vi "SUB_WriteFileAppendText_AnyFolder.vi"(2 "Input Text":string, 3 "Filename":string, 4 "base path":path) -> ()   [LabVIEW 2011]
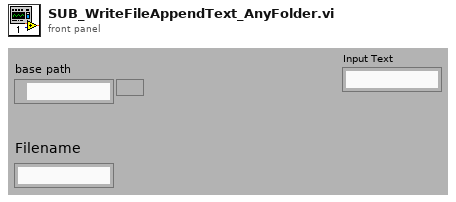
[diagram p1: front panel]
types:
  T1 = enum16{"open", "open or create", "create or replace", "create", "open (read only)"}
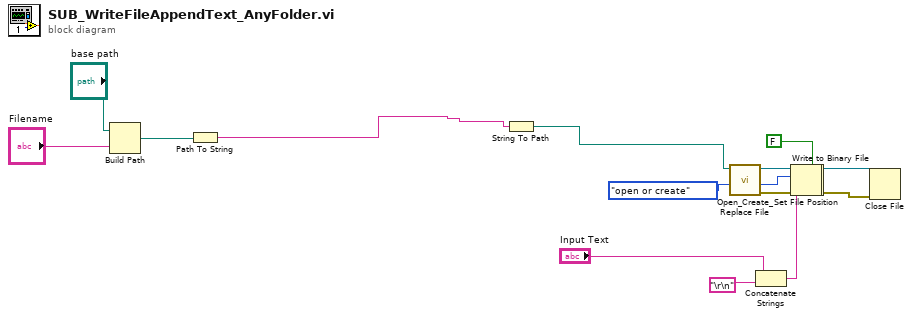
[diagram p0: block diagram]
diagram:
  n1 = Build Path(base path="base path", name or relative path="Filename") -> (appended path=w6:path)
  n2 = Path To String(path=w6) -> (string=w5:string)
  n3 = String To Path(string=w5) -> (path=w2:path)
  n4 = call <vilib>:"Open_Create_Replace File.vi"("function (open:0)"=T1."open or create", "file path"=w2) -> ("error out"=w16:errorcluster, "file size (bytes)"=w14:i32, "refnum"=w15:refnum<file>)  [unwired: 6 in, 1 out]
  n5 = Concatenate Strings("Input Text", "\r\n") -> (w10:string)
  n6 = Set File Position(offset (in bytes) (0)=w14, refnum=w15, error in=w16) -> (refnum out=w9:refnum<file>, error out=w8:errorcluster)  [unwired: 1 in]
  n7 = Write to Binary File(file (use dialog)=w9, data=w10, error in=w8, 5:FALSE ("prepend array or string size? (T)")) -> (refnum out=w12:refnum<file>, error out=w13:errorcluster)  [unwired: 2 in, 1 out]
  n8 = Close File(refnum=w12, error in=w13) -> ()  [unwired: 2 out]
